vi "DAQ-PXIe_DataControlArrayConfigs.vi"(8 "error in":errorcluster, 9 "DAQmx Cluster In":T2 {"ai DAQmx Cluster"."input terminal configuration" items=["Default"=-1, "RSE"=10083, "NRSE"=10078, "Differential"=10106, "Pseudodifferential"=12529]; "bc DAQmx Cluster"."Scaling Information"."electrical units" items=["Volts/Volt"=15896, "mVolts/Volt"=15897]; "bc DAQmx Cluster"."Scaling Information"."physical units" items=["Newtons"=15875, "Pounds"=15876, "kgf"=15877]; "bc DAQmx Cluster"."Bridge Information"."bridge configuration" items=["Full Bridge"=10182, "Half Bridge"=10187, "Quarter Bridge"=10270]; "bc DAQmx Cluster"."Bridge Information"."voltage excitation source" items=["Internal"=10200, "External"=10167]; "tc DAQmx Cluster"."Thermocouple Type" items=["J"=10072, "K"=10073, "N"=10077, "R"=10082, "S"=10085, "T"=10086, "B"=10047, "E"=10055]; "tc DAQmx Cluster"."Units" items=["Deg C"=10143, "Deg F"=10144, "Kelvins"=10325, "Deg R"=10145, "From Custom Scale"=10065]}, 10 "Calibration Configuration In":T3, 11 "StreamCluster_TypeDef":T1) -> (0 "error out":errorcluster={"status"=TRUE, "code"=0, "source"=""}, 1 "DAQmx Cluster Out":T2 {"ai DAQmx Cluster"."input terminal configuration" items=["Default"=-1, "RSE"=10083, "NRSE"=10078, "Differential"=10106, "Pseudodifferential"=12529]; "bc DAQmx Cluster"."Scaling Information"."electrical units" items=["Volts/Volt"=15896, "mVolts/Volt"=15897]; "bc DAQmx Cluster"."Scaling Information"."physical units" items=["Newtons"=15875, "Pounds"=15876, "kgf"=15877]; "bc DAQmx Cluster"."Bridge Information"."bridge configuration" items=["Full Bridge"=10182, "Half Bridge"=10187, "Quarter Bridge"=10270]; "bc DAQmx Cluster"."Bridge Information"."voltage excitation source" items=["Internal"=10200, "External"=10167]; "tc DAQmx Cluster"."Thermocouple Type" items=["J"=10072, "K"=10073, "N"=10077, "R"=10082, "S"=10085, "T"=10086, "B"=10047, "E"=10055]; "tc DAQmx Cluster"."Units" items=["Deg C"=10143, "Deg F"=10144, "Kelvins"=10325, "Deg R"=10145, "From Custom Scale"=10065]}, 2 "Calibration Configuration Out":T3)   [LabVIEW 2024]
uses:
  <vilib>/ErrorRing/Error Ring.xnode
  <vilib>/Utility/error.llb/Error Cluster From Error Code.vi
  Configuration/Calibration Configuration.ctl
  Configuration/DAQmx Configuration.ctl
  Control/StreamCluster_TypeDef.ctl
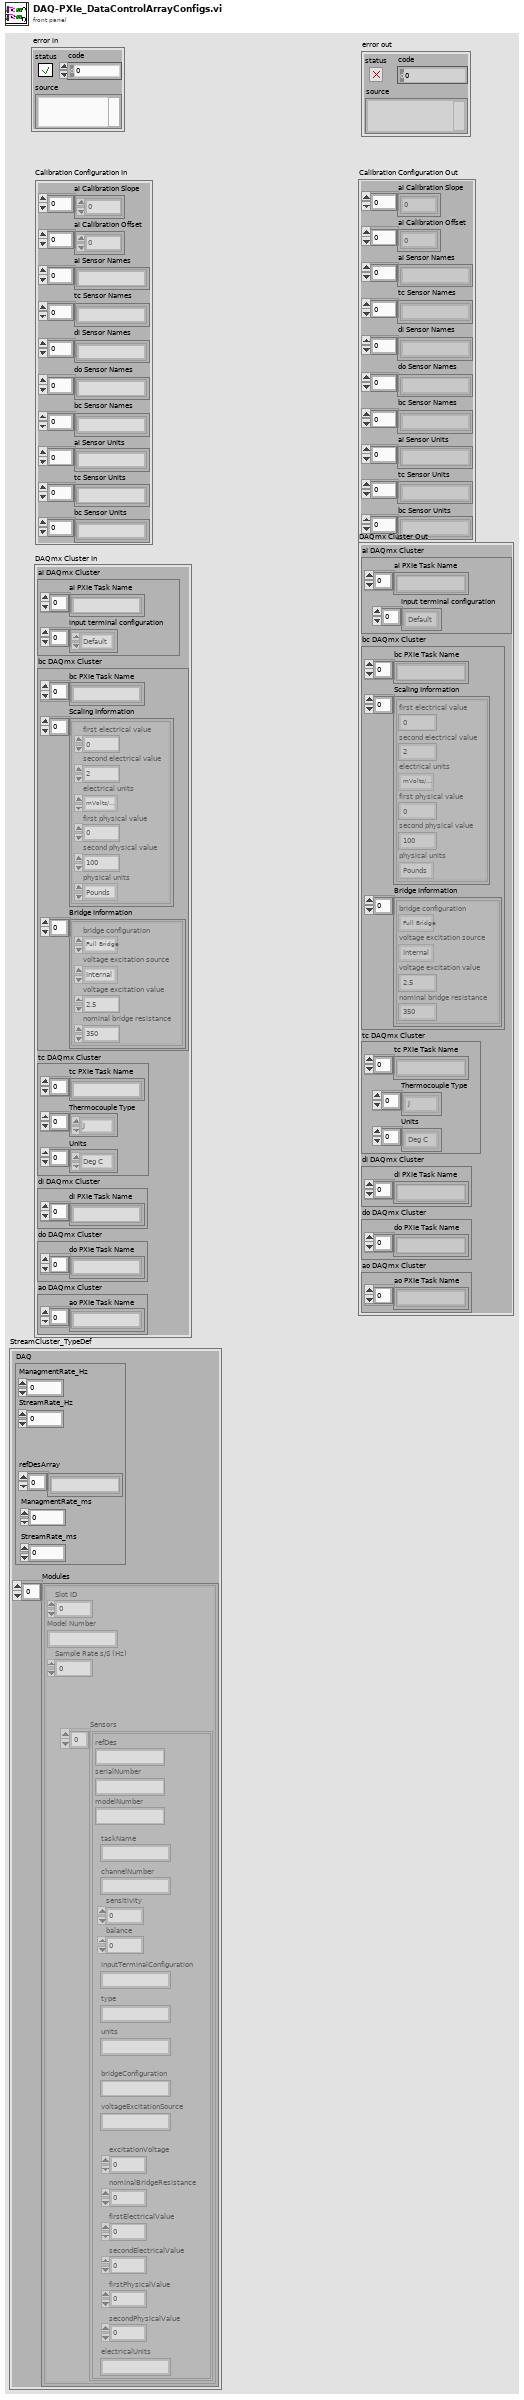
[diagram p1: front panel]
types:
  T1 = typedef "StreamCluster_TypeDef.ctl" = cluster{"DAQ":cluster{"ManagmentRate_Hz":i32, "StreamRate_Hz":i32, "refDesArray":string[], "StreamRate_ms":i32, "ManagmentRate_ms":i32}, "Modules":cluster{"Slot ID":i32, "Model Number":string, "Sample Rate s/S (Hz)":dbl, "Sensors":cluster{"refDes":string, "serialNumber":string, "modelNumber":string, "units":string, "balance":dbl, "sensitivity":dbl, "type":string, "inputTerminalConfiguration":string, "channelNumber":string, "taskName":string, "bridgeConfiguration":string, "excitationVoltage":dbl, "voltageExcitationSource":string, "nominalBridgeResistance":dbl, "firstElectricalValue":dbl, "secondElectricalValue":dbl, "firstPhysicalValue":dbl, "secondPhysicalValue":dbl, "electricalUnits":string}[]}[]}
  T2 = typedef "DAQmx Configuration.ctl" = cluster{"ai DAQmx Cluster":cluster{"ai PXIe Task Name":string[], "input terminal configuration":i32[]}, "bc DAQmx Cluster":cluster{"bc PXIe Task Name":string[], "Scaling Information":cluster{"first electrical value":dbl, "second electrical value":dbl, "electrical units":i32, "first physical value":dbl, "second physical value":dbl, "physical units":i32}[], "Bridge Information":cluster{"bridge configuration":i32, "voltage excitation source":i32, "voltage excitation value":dbl, "nominal bridge resistance":dbl}[]}, "tc DAQmx Cluster":cluster{"tc PXIe Task Name":string[], "Thermocouple Type":i32[], "Units":i32[]}, "di DAQmx Cluster":cluster{"di PXIe Task Name":string[]}, "do DAQmx Cluster":cluster{"do PXIe Task Name":string[]}, "ao DAQmx Cluster":cluster{"ao PXIe Task Name":string[]}}
  T3 = typedef "Calibration Configuration.ctl" = cluster{"ai Calibration Slope":dbl[], "ai Calibration Offset":dbl[], "ai Sensor Names ":string[], "tc Sensor Names":string[], "di Sensor Names":string[], "do Sensor Names":string[], "bc Sensor Names":string[], "ai Sensor Units":string[], "tc Sensor Units":string[], "bc Sensor Units":string[]}
  T4 = cluster{"bridge configuration":i32, "voltage excitation source":i32, "voltage excitation value":dbl, "nominal bridge resistance":dbl}
  T5 = cluster{"first electrical value":dbl, "second electrical value":dbl, "electrical units":i32, "first physical value":dbl, "second physical value":dbl, "physical units":i32}
  T6 = cluster{"Slot ID":i32, "Model Number":string, "Sample Rate s/S (Hz)":dbl, "Sensors":cluster{"refDes":string, "serialNumber":string, "modelNumber":string, "units":string, "balance":dbl, "sensitivity":dbl, "type":string, "inputTerminalConfiguration":string, "channelNumber":string, "taskName":string, "bridgeConfiguration":string, "excitationVoltage":dbl, "voltageExcitationSource":string, "nominalBridgeResistance":dbl, "firstElectricalValue":dbl, "secondElectricalValue":dbl, "firstPhysicalValue":dbl, "secondPhysicalValue":dbl, "electricalUnits":string}[]}[]
  T7 = cluster{"refDes":string, "serialNumber":string, "modelNumber":string, "units":string, "balance":dbl, "sensitivity":dbl, "type":string, "inputTerminalConfiguration":string, "channelNumber":string, "taskName":string, "bridgeConfiguration":string, "excitationVoltage":dbl, "voltageExcitationSource":string, "nominalBridgeResistance":dbl, "firstElectricalValue":dbl, "secondElectricalValue":dbl, "firstPhysicalValue":dbl, "secondPhysicalValue":dbl, "electricalUnits":string}[]
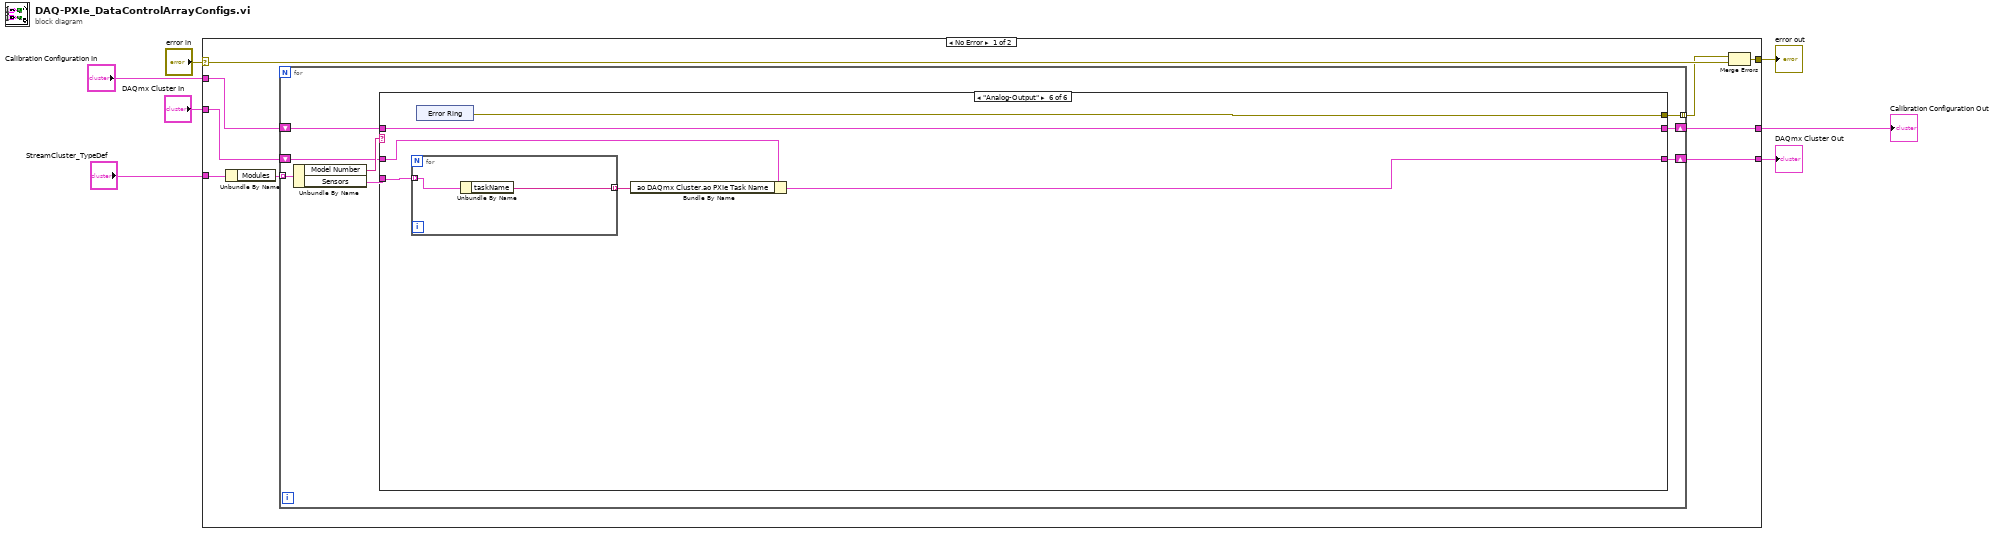
[diagram p0: block diagram]
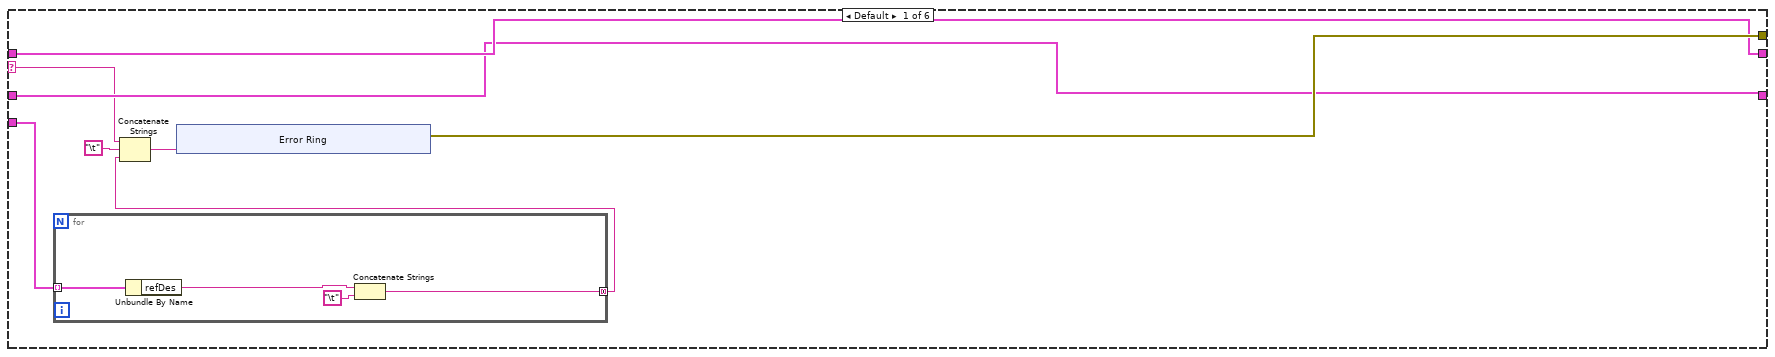
[diagram p2: hidden frame]
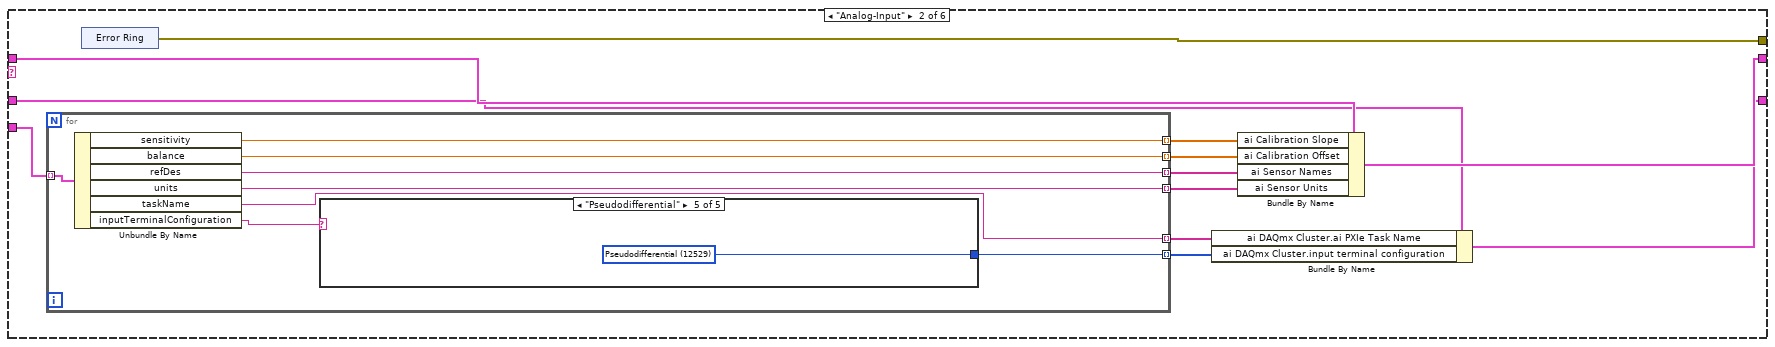
[diagram p3: hidden frame]
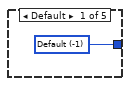
[diagram p4: hidden frame]
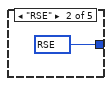
[diagram p5: hidden frame]
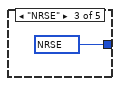
[diagram p6: hidden frame]
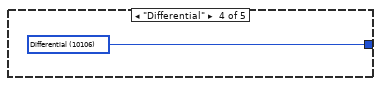
[diagram p7: hidden frame]
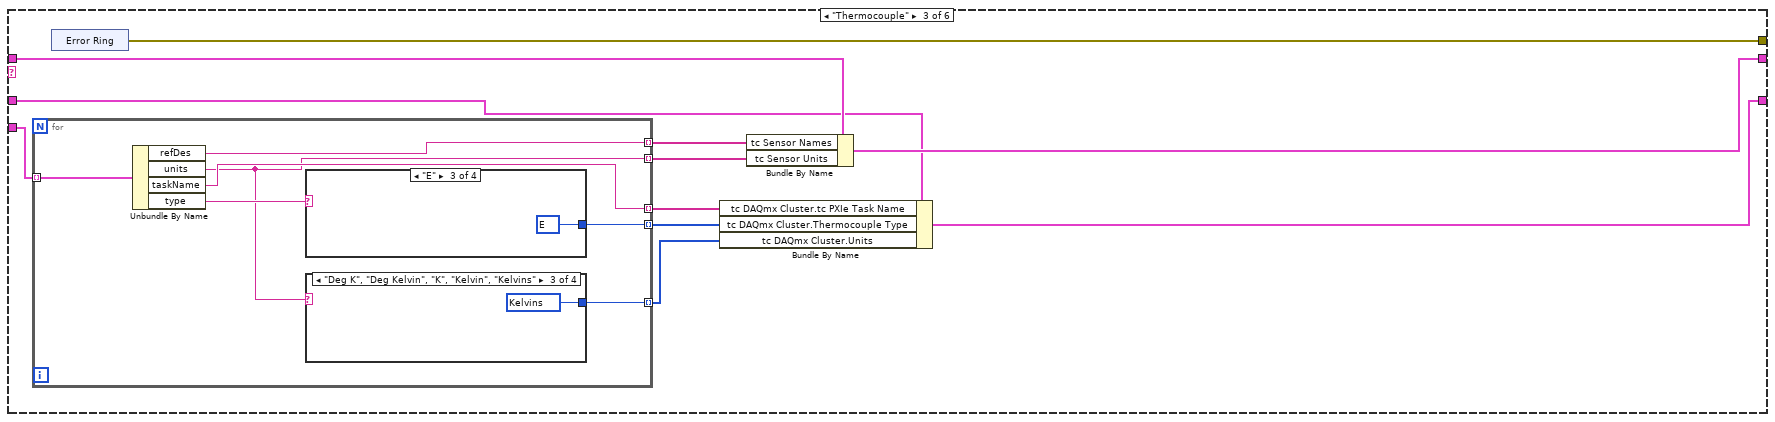
[diagram p8: hidden frame]
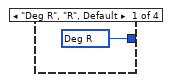
[diagram p9: hidden frame]
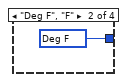
[diagram p10: hidden frame]
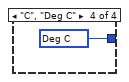
[diagram p11: hidden frame]
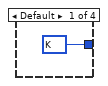
[diagram p12: hidden frame]
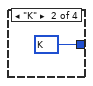
[diagram p13: hidden frame]
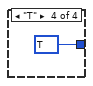
[diagram p14: hidden frame]
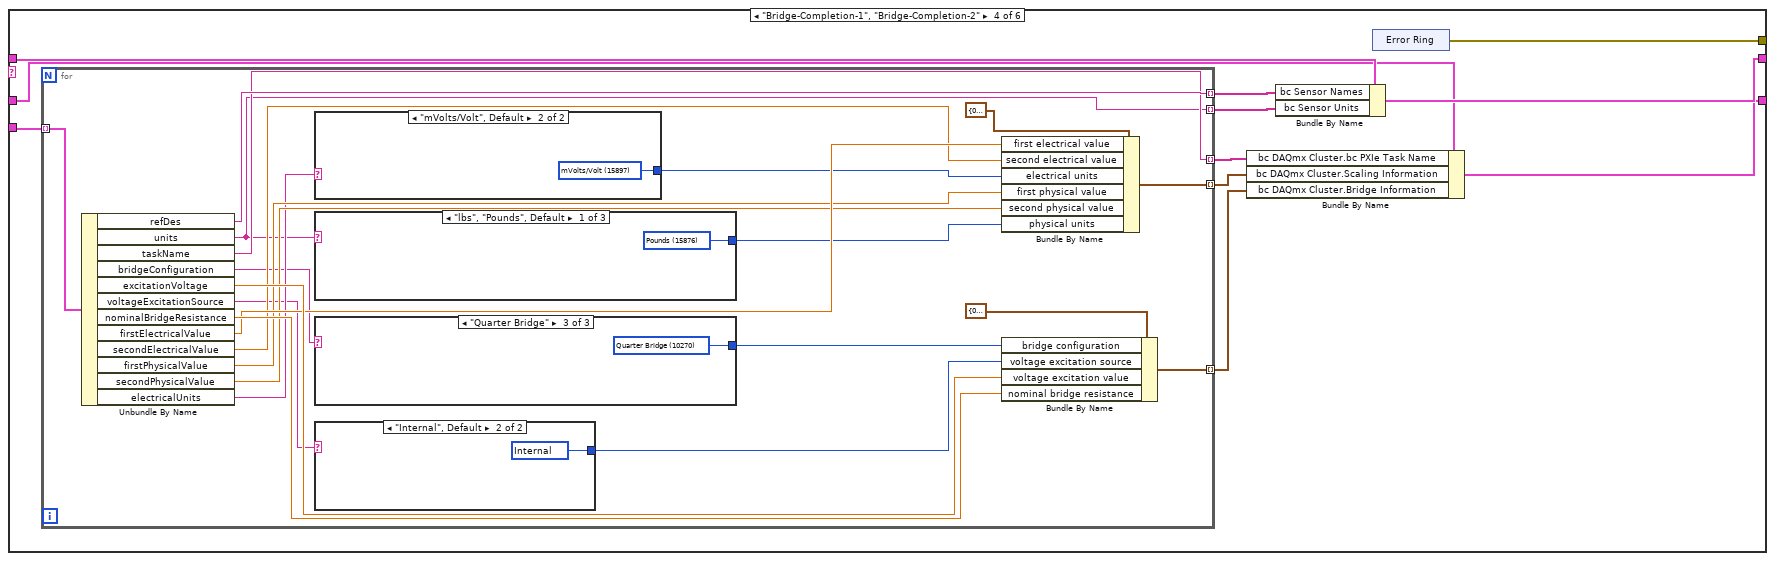
[diagram p15: hidden frame]
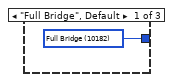
[diagram p16: hidden frame]
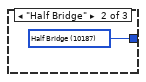
[diagram p17: hidden frame]
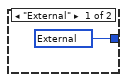
[diagram p18: hidden frame]
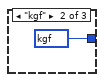
[diagram p19: hidden frame]
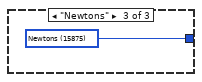
[diagram p20: hidden frame]
diagram:
  n1 = case shown="No Error" "error in" {
    selector: "error in" -> [w13 w176]
    tunnel: [w14 w176] -> w6
    tunnel: "StreamCluster_TypeDef" -> [w16 _]
    tunnel: [w12 w175] -> w5
    tunnel: "Calibration Configuration In" -> [w15 w175]
    tunnel: [w10 w174] -> w3
    tunnel: "DAQmx Cluster In" -> [w11 w174]
    frame No Error {
      n2 = Unbundle By Name(w16) -> ("Modules"=w9:T6)
      n3 = for {
        tunnel: w9 -> [w23] mode=indexing
        shift-right: [w20] -> w12
        shift-left: w15 -> [w22]
        tunnel: [w19] -> w8 mode=indexing
        shift-right: [w17] -> w10
        shift-left: w11 -> [w18]
        n4 = Unbundle By Name(w23) -> ("Model Number"=w24:string, "Sensors"=w21:T7)
        n5 = case shown="\"Analog-Output\"" w24 {
          selector: w24 -> [w27 _ _ _ _ _]
          tunnel: w22 -> [w31 w55 w79 w106 w149 w166]
          tunnel: w21 -> [w29 w54 w78 w105 w151 w170]
          tunnel: [w31 w49 w80 w107 w147 w166] -> w20
          tunnel: [w32 w48 w75 w102 w150 w169] -> w19
          tunnel: w18 -> [w30 w47 w74 w101 w144 w168]
          tunnel: [w30 w44 w73 w97 w140 w165] -> w17
          frame Default {
            n6 = for {
              tunnel: w29 -> [w36] mode=indexing
              tunnel: [w33] -> w28 mode=concatenating
              n7 = Unbundle By Name(w36) -> ("refDes"=w35:string)
              n8 = Concatenate Strings(w35, "\t") -> (w33:string)
            }
            n9 = Concatenate Strings(w27, "\t", w28) -> (w25:string)
            n10 = xnode "Error Ring"("parameter 0"=w25) -> ("error out"=w32:errorcluster)
          }
          frame "Analog-Input" {
            n11 = for {
              tunnel: w54 -> [w64] mode=indexing
              tunnel: [w63] -> w53 mode=indexing
              tunnel: [w62] -> w52 mode=indexing
              tunnel: [w61] -> w51 mode=indexing
              tunnel: [w60] -> w50 mode=indexing
              tunnel: [w59] -> w46 mode=indexing
              tunnel: [w57] -> w45 mode=indexing
              n12 = Unbundle By Name(w64) -> ("sensitivity"=w63:dbl, "balance"=w62:dbl, "refDes"=w61:string, "units"=w60:string, "taskName"=w59:string, "inputTerminalConfiguration"=w58:string)
              n13 = case shown="\"Pseudodifferential\"" w58 {
                tunnel: [w65 w66 w67 w68 w69] -> w57
                frame Default {
                  w65 = -1 items=["Default"=-1, "RSE"=10083, "NRSE"=10078, "Differential"=10106, "Pseudodifferential"=12529] ("input terminal configuration")
                }
                frame "RSE" {
                  w66 = 10083 items=["Default"=-1, "RSE"=10083, "NRSE"=10078, "Differential"=10106, "Pseudodifferential"=12529] ("input terminal configuration")
                }
                frame "NRSE" {
                  w67 = 10078 items=["Default"=-1, "RSE"=10083, "NRSE"=10078, "Differential"=10106, "Pseudodifferential"=12529] ("input terminal configuration")
                }
                frame "Differential" {
                  w68 = 10106 items=["Default"=-1, "RSE"=10083, "NRSE"=10078, "Differential"=10106, "Pseudodifferential"=12529] ("input terminal configuration")
                }
                frame "Pseudodifferential" {
                  w69 = 12529 items=["Default"=-1, "RSE"=10083, "NRSE"=10078, "Differential"=10106, "Pseudodifferential"=12529] ("input terminal configuration")
                }
              }
            }
            n14 = xnode "Error Ring"() -> ("error out"=w48:errorcluster)
            n15 = Bundle By Name(cluster=w47, "ai DAQmx Cluster.ai PXIe Task Name"=w46, "ai DAQmx Cluster.input terminal configuration"=w45) -> (w44:T2)
            n16 = Bundle By Name(cluster=w55, "ai Calibration Slope"=w53, "ai Calibration Offset"=w52, "ai Sensor Names"=w51, "ai Sensor Units"=w50) -> (w49:T3)
          }
          frame "Thermocouple" {
            n17 = for {
              tunnel: w78 -> [w88] mode=indexing
              tunnel: [w87] -> w77 mode=indexing
              tunnel: [w83] -> w76 mode=indexing
              tunnel: [w86] -> w72 mode=indexing
              tunnel: [w84] -> w71 mode=indexing
              tunnel: [w82] -> w70 mode=indexing
              n18 = Unbundle By Name(w88) -> ("refDes"=w87:string, "units"=w83:string, "taskName"=w86:string, "type"=w85:string)
              n19 = case shown="\"E\"" w85 {
                tunnel: [w93 w94 w95 w96] -> w84
                frame Default {
                  w93 = 10073 items=["J"=10072, "K"=10073, "N"=10077, "R"=10082, "S"=10085, "T"=10086, "B"=10047, "E"=10055] ("thermocouple type")
                }
                frame "K" {
                  w94 = 10073 items=["J"=10072, "K"=10073, "N"=10077, "R"=10082, "S"=10085, "T"=10086, "B"=10047, "E"=10055] ("thermocouple type")
                }
                frame "E" {
                  w95 = 10055 items=["J"=10072, "K"=10073, "N"=10077, "R"=10082, "S"=10085, "T"=10086, "B"=10047, "E"=10055] ("thermocouple type")
                }
                frame "T" {
                  w96 = 10086 items=["J"=10072, "K"=10073, "N"=10077, "R"=10082, "S"=10085, "T"=10086, "B"=10047, "E"=10055] ("thermocouple type")
                }
              }
              n20 = case shown="\"Deg K\", \"Deg Kelvin\", \"K\", \"Kelvin\", \"Kelvins\"" w83 {
                tunnel: [w89 w90 w91 w92] -> w82
                frame "Deg R", "R", Default {
                  w89 = 10145 items=["Deg C"=10143, "Deg F"=10144, "Kelvins"=10325, "Deg R"=10145, "From Custom Scale"=10065] ("units")
                }
                frame "Deg F", "F" {
                  w90 = 10144 items=["Deg C"=10143, "Deg F"=10144, "Kelvins"=10325, "Deg R"=10145, "From Custom Scale"=10065] ("units")
                }
                frame "Deg K", "Deg Kelvin", "K", "Kelvin", "Kelvins" {
                  w91 = 10325 items=["Deg C"=10143, "Deg F"=10144, "Kelvins"=10325, "Deg R"=10145, "From Custom Scale"=10065] ("units")
                }
                frame "C", "Deg C" {
                  w92 = 10143 items=["Deg C"=10143, "Deg F"=10144, "Kelvins"=10325, "Deg R"=10145, "From Custom Scale"=10065] ("units")
                }
              }
            }
            n21 = xnode "Error Ring"() -> ("error out"=w75:errorcluster)
            n22 = Bundle By Name(cluster=w74, "tc DAQmx Cluster.tc PXIe Task Name"=w72, "tc DAQmx Cluster.Thermocouple Type"=w71, "tc DAQmx Cluster.Units"=w70) -> (w73:T2)
            n23 = Bundle By Name(cluster=w79, "tc Sensor Names"=w77, "tc Sensor Units"=w76) -> (w80:T3)
          }
          frame "Bridge-Completion-1", "Bridge-Completion-2" {
            n24 = for {
              tunnel: w105 -> [w129] mode=indexing
              tunnel: [w128] -> w104 mode=indexing
              tunnel: [w114] -> w103 mode=indexing
              tunnel: [w127] -> w100 mode=indexing
              tunnel: [w126] -> w99 mode=indexing
              tunnel: [w124] -> w98 mode=indexing
              n25 = Unbundle By Name(w129) -> ("refDes"=w128:string, "units"=w114:string, "taskName"=w127:string, "bridgeConfiguration"=w110:string, "excitationVoltage"=w122:dbl, "voltageExcitationSource"=w112:string, "nominalBridgeResistance"=w121:dbl, "firstElectricalValue"=w120:dbl, "secondElectricalValue"=w119:dbl, "firstPhysicalValue"=w118:dbl, "secondPhysicalValue"=w117:dbl, "electricalUnits"=w116:string)
              n26 = case shown="\"mVolts/Volt\", Default" w116 {
                tunnel: [w138 w139] -> w115
                frame "Volts/Volt" {
                  w138 = 15896 items=["Volts/Volt"=15896, "mVolts/Volt"=15897] ("electrical units")
                }
                frame "mVolts/Volt", Default {
                  w139 = 15897 items=["Volts/Volt"=15896, "mVolts/Volt"=15897] ("electrical units")
                }
              }
              n27 = case shown="\"lbs\", \"Pounds\", Default" w114 {
                tunnel: [w135 w136 w137] -> w113
                frame "lbs", "Pounds", Default {
                  w135 = 15876 items=["Newtons"=15875, "Pounds"=15876, "kgf"=15877] ("physical units")
                }
                frame "kgf" {
                  w136 = 15877 items=["Newtons"=15875, "Pounds"=15876, "kgf"=15877] ("physical units")
                }
                frame "Newtons" {
                  w137 = 15875 items=["Newtons"=15875, "Pounds"=15876, "kgf"=15877] ("physical units")
                }
              }
              n28 = case shown="\"Quarter Bridge\"" w110 {
                tunnel: [w130 w131 w132] -> w109
                frame "Full Bridge", Default {
                  w130 = 10182 items=["Full Bridge"=10182, "Half Bridge"=10187, "Quarter Bridge"=10270] ("bridge configuration")
                }
                frame "Half Bridge" {
                  w131 = 10187 items=["Full Bridge"=10182, "Half Bridge"=10187, "Quarter Bridge"=10270] ("bridge configuration")
                }
                frame "Quarter Bridge" {
                  w132 = 10270 items=["Full Bridge"=10182, "Half Bridge"=10187, "Quarter Bridge"=10270] ("bridge configuration")
                }
              }
              n29 = case shown="\"Internal\", Default" w112 {
                tunnel: [w133 w134] -> w111
                frame "External" {
                  w133 = 10167 items=["Internal"=10200, "External"=10167] ("voltage excitation source")
                }
                frame "Internal", Default {
                  w134 = 10200 items=["Internal"=10200, "External"=10167] ("voltage excitation source")
                }
              }
              n30 = Bundle By Name(cluster=T5 {"first electrical value"=0.0, "second electrical value"=0.0, "electrical units"=0, "first physical value"=0.0, "second physical value"=0.0, "physical units"=0} ("scaling information"), "first electrical value"=w120, "second electrical value"=w119, "electrical units"=w115, "first physical value"=w118, "second physical value"=w117, "physical units"=w113) -> (w126:T5)
              n31 = Bundle By Name(cluster=T4 {"bridge configuration"=0, "voltage excitation source"=0, "voltage excitation value"=0.0, "nominal bridge resistance"=0.0} ("bridge information"), "bridge configuration"=w109, "voltage excitation source"=w111, "voltage excitation value"=w122, "nominal bridge resistance"=w121) -> (w124:T4)
            }
            n32 = Bundle By Name(cluster=w101, "bc DAQmx Cluster.bc PXIe Task Name"=w100, "bc DAQmx Cluster.Scaling Information"=w99, "bc DAQmx Cluster.Bridge Information"=w98) -> (w97:T2)
            n33 = Bundle By Name(cluster=w106, "bc Sensor Names"=w104, "bc Sensor Units"=w103) -> (w107:T3)
            n34 = xnode "Error Ring"() -> ("error out"=w102:errorcluster)
          }
          frame "Digital-IO" {
            n35 = for {
              tunnel: w151 -> [w164] mode=indexing
              tunnel: [w163] -> w145 mode=indexing if=w155
              tunnel: [w163] -> w146 mode=indexing if=w157
              tunnel: [w156] -> w143 mode=indexing if=w157
              tunnel: [w156] -> w141 mode=indexing if=w155
              n36 = Unbundle By Name(w164) -> ("refDes"=w163:string, "taskName"=w156:string)
              n37 = String Length(string=w156) -> (length=w161:i32)
              n38 = Subtract(x=w161, y=7) -> (x-y=w159:i32)
              n39 = String Subset(string=w156, offset (0)=w159, length (rest)=1 ("length (rest)")) -> (substring=w158:string)
              n40 = Decimal String To Number(string=w158) -> (number=w154:i32)  [unwired: 2 in, 1 out]
              n41 = Greater?(x=w154, y=2 ("x")) -> (0:w155:bool)
              n42 = Not(x=w155) -> (.not. x?=w157:bool)
            }
            n43 = Bundle By Name(cluster=w144, "di DAQmx Cluster.di PXIe Task Name"=w143) -> (w142:T2)
            n44 = Bundle By Name(cluster=w149, "di Sensor Names"=w146) -> (w148:T3)
            n45 = Bundle By Name(cluster=w142, "do DAQmx Cluster.do PXIe Task Name"=w141) -> (w140:T2)
            n46 = Bundle By Name(cluster=w148, "do Sensor Names"=w145) -> (w147:T3)
            n47 = xnode "Error Ring"() -> ("error out"=w150:errorcluster)
          }
          frame "Analog-Output" {
            n48 = for {
              tunnel: w170 -> [w173] mode=indexing
              tunnel: [w172] -> w167 mode=indexing
              n49 = Unbundle By Name(w173) -> ("taskName"=w172:string)
            }
            n50 = xnode "Error Ring"() -> ("error out"=w169:errorcluster)
            n51 = Bundle By Name(cluster=w168, "ao DAQmx Cluster.ao PXIe Task Name"=w167) -> (w165:T2)
          }
        }
      }
      n52 = Merge Errors(w8, w13) -> (w14:errorcluster)
    }
    frame Error {
    }
  }
  "error out" <- w6
  "Calibration Configuration Out" <- w5
  "DAQmx Cluster Out" <- w3
